vi "Initialize.vi"(8 "error in (no error)":errorcluster, 9 "Reset (T: Enabled)":bool=TRUE, 10 "ID Query (T: Enabled)":bool=TRUE, 11 "VISA resource name":refnum<visa-resource-name>) -> (0 "error out":errorcluster, 3 "VISA resource name out":refnum<visa-resource-name>)   [LabVIEW 2021, in "Sorensen M9A Series.lvlib"]
doc: "This VI passes the addressing information in the instrument descriptor. It can check the instrument ID to make sure the contacted instrument is whichever power supply that is being used via the \"ID?\" querry, but the user will need to know the proper string that the device returns from such a querry. At this time, only the DLM 8-75 power supply's ID string is known to the author. If the ID String terminal is left unwired, the ID Querry terminal should be wired to a \"false\" constant.\nAdditionally, the power supply can be reset to its default on condition."
uses:
  Sorensen M9A Series.lvlib
panel:
  # "(c) 2004-2009 National Instruments.  ALL RIGHTS RESERVED."
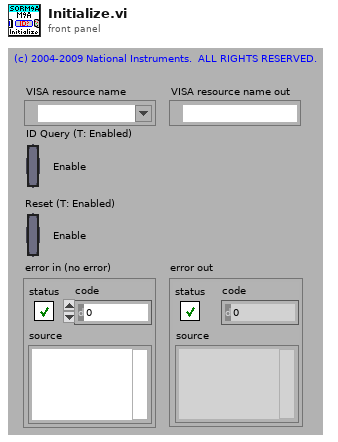
[diagram p1: front panel]
types:
  T1 = cluster{"Status":bool, "Code":i32, "Source (VI Name)":string}
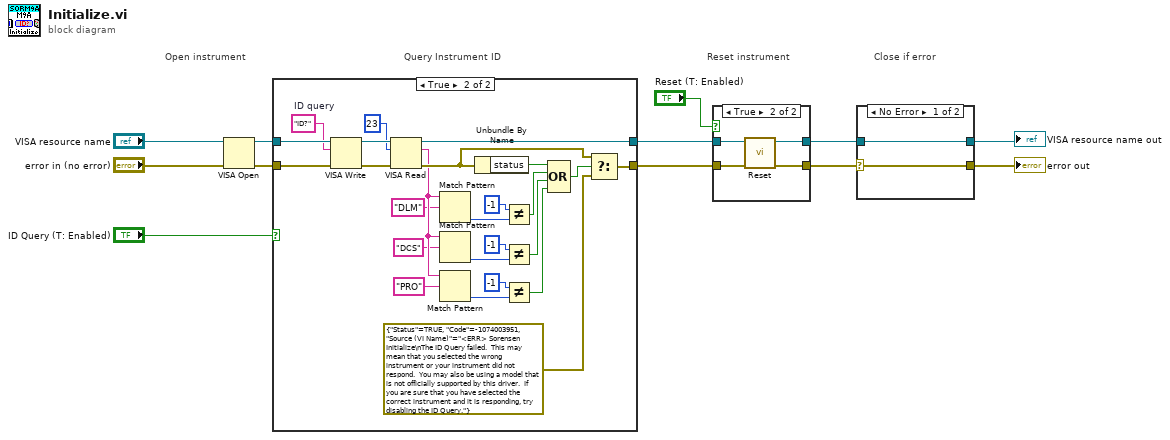
[diagram p0: block diagram]
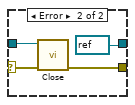
[diagram p2: hidden frame]
diagram:
  # "Close if error"
  # "Query Instrument ID"
  # "Reset instrument"
  # "Open instrument"
  n1 = VISA Open(error in (no error)="error in (no error)", VISA resource name="VISA resource name") -> (VISA resource name=w8:refnum<visa-resource-name>, error out=w7:errorcluster)  [unwired: 3 in]
  n2 = case shown="True" "ID Query (T: Enabled)" {
    tunnel: [w13 w39] -> w10
    tunnel: [w14 w36] -> w11
    tunnel: w8 -> [w14 w37]
    tunnel: w7 -> [w13 w38]
    frame False {
    }
    frame True {
      w35 = "ID?"  # ID query
      n3 = VISA Write(VISA resource name=w37, write buffer=w35, error in (no error)=w38) -> (VISA resource name out=w29:refnum<visa-resource-name>, error out=w30:errorcluster)  [unwired: 1 out]
      n4 = VISA Read(VISA resource name=w29, byte count=u32 23, error in (no error)=w30) -> (VISA resource name out=w36:refnum<visa-resource-name>, read buffer=w25:string, error out=w27:errorcluster)  [unwired: 1 out]
      n5 = Match Pattern(string=w25, regular expression="DLM") -> (offset past match=w34:i32)  [unwired: 1 in, 3 out]
      n6 = Match Pattern(string=w25, regular expression="DCS") -> (offset past match=w21:i32)  [unwired: 1 in, 3 out]
      n7 = Match Pattern(string=w25, regular expression="PRO") -> (offset past match=w22:i32)  [unwired: 1 in, 3 out]
      n8 = Unbundle By Name(w27) -> ("status"=w32:bool)
      n9 = Not Equal?(x=-1, y=w34) -> (x != y?=w28:bool)
      n10 = Not Equal?(x=-1, y=w21) -> (x != y?=w20:bool)
      n11 = Not Equal?(x=-1, y=w22) -> (x != y?=w19:bool)
      n12 = Compound Arithmetic op=OR(w32, w28, w20, w19) -> (w31:bool)
      n13 = Select(t=w27, s=w31, f=T1 {"Status"=TRUE, "Code"=-1074003951, "Source (VI Name)"="<ERR> Sorensen Initialize\nThe ID Query failed.  This may mean that you selected the wrong instrument or your instrument did not respond.  You may also be using a model that is not officially supported by this driver.  If you are sure that you have selected the correct instrument and it is responding, try disabling the ID Query."}) -> (s? t:f=w39:T1)
    }
  }
  n14 = case shown="True" "Reset (T: Enabled)" {
    tunnel: w10 -> [w41 w44]
    tunnel: [w41 w42] -> w4
    tunnel: w11 -> [w40 w45]
    tunnel: [w40 w43] -> w3
    frame False {
    }
    frame True {
      n15 = call "Reset.vi"("error in (no error)"=w44, "VISA resource name"=w45) -> ("error out"=w42:errorcluster, "VISA resource name out"=w43:refnum<visa-resource-name>)  [unwired: 8 in]
    }
  }
  n16 = case shown="No Error" w4 {
    selector: w4 -> [w47 w49]
    tunnel: w3 -> [w46 w50]
    tunnel: [w47 w48] -> w2
    tunnel: [w46 refnum<visa-resource-name> refnum ("VISA resource name 2")] -> w1
    frame No Error {
    }
    frame Error {
      n17 = call "Close.vi"("error in (no error)"=w49, "VISA resource name"=w50) -> ("error out"=w48:errorcluster)  [unwired: 9 in]
    }
  }
  "error out" <- w2
  "VISA resource name out" <- w1
